vi "Comm_Vars.vi"() -> ()   [LabVIEW 2010]
uses:
  Ctrls/Main_Msg_type.ctl
panel:
  in  "Main queue":refnum<queue>
  in  "Comm_Vars":T1(array[cluster])
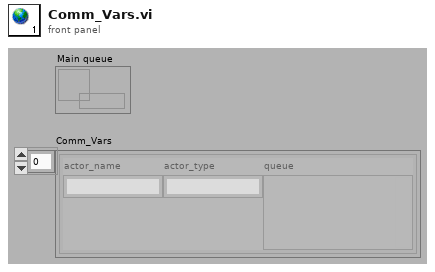
[diagram p1: front panel]
types:
  T1 = cluster{"actor_name":string, "actor_type":string, "queue":variant}[]
diagram:
